vi "20TILM_Merge_Cluster.vi"(1 "20TILM Control":T3, 2 "20TILM Status":T1) -> (0 "20TILM Cluster":T2)   [LabVIEW 2019]
uses:
  Gustav/20TILM_Control.ctl
  Gustav/20TILM_Cluster.ctl
  Gustav/20TILM_Status.ctl
panel:
  # "Levelmeter"
  # "Helium (%)"
  # "Levelmeter"
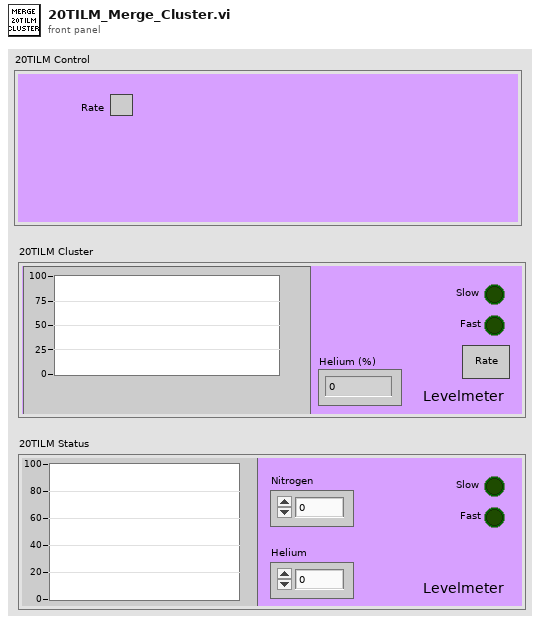
[diagram p1: front panel]
types:
  T1 = typedef "20TILM_Status.ctl" = cluster{"Helium":dbl, "Nitrogen":dbl, "Slow":bool, "Fast":bool, "Plot":cluster{"X":dbl, "Y":dbl}[]}
  T2 = typedef "20TILM_Cluster.ctl" = cluster{"Helium":dbl, "Nitrogen":dbl, "Slow":bool, "Fast":bool, "Plot":cluster{"X":dbl, "Y":dbl}[], "Rate":bool}
  T3 = typedef "20TILM_Control.ctl" = cluster{"Rate":bool}
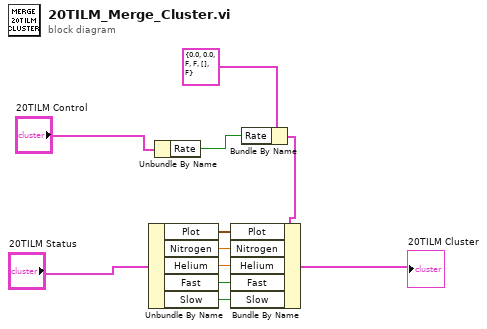
[diagram p0: block diagram]
diagram:
  n1 = Unbundle By Name("20TILM Status") -> ("Plot"=w11:cluster{"X":dbl, "Y":dbl}[], "Nitrogen"=w10:dbl, "Helium"=w9:dbl, "Fast"=w8:bool, "Slow"=w7:bool)
  n2 = Unbundle By Name("20TILM Control") -> ("Rate"=w6:bool)
  n3 = Bundle By Name(cluster=T2 {"Helium"=0.0, "Nitrogen"=0.0, "Slow"=FALSE, "Fast"=FALSE, "Plot"=[], "Rate"=FALSE} ("20TILM"), "Rate"=w6) -> (w5:T2)
  n4 = Bundle By Name(cluster=w5, "Plot"=w11, "Nitrogen"=w10, "Helium"=w9, "Fast"=w8, "Slow"=w7) -> (→"20TILM Cluster":T2)
